vi "Read Static Values.vi"(8 "error in (no error)":errorcluster, 10 "Measurement (0: Current)":u16(ring) items=["Current", "Voltage", "Resistance", "Power", "Temperature", "MPPT Energy"], 11 "VISA resource name":refnum<visa-resource-name>) -> (0 "error out":errorcluster, 2 "Measurement":dbl format="%^#_6g", 3 "VISA resource name out":refnum<visa-resource-name>)   [LabVIEW 2021, in "HH PLI Series.lvlib"]
doc: "Reads static values of current, voltage, resistance, power, instrument temperature and MPPT energy."
uses:
  HH PLI Series.lvlib
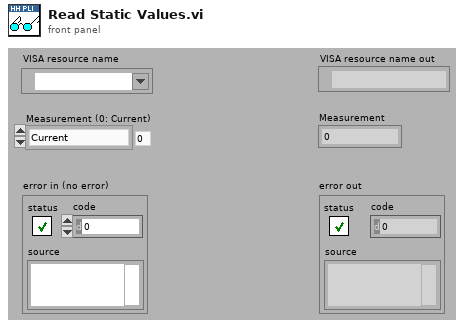
[diagram p1: front panel]
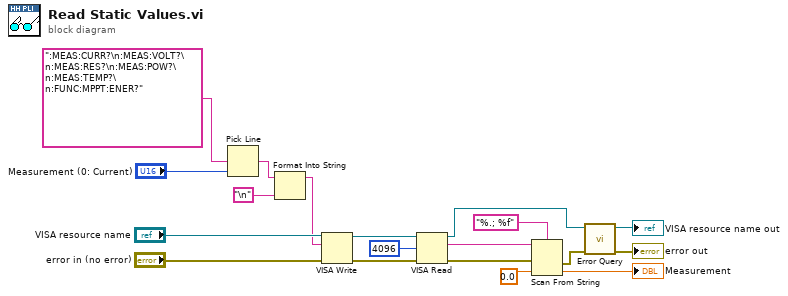
[diagram p0: block diagram]
diagram:
  n1 = Pick Line(multi-line string=":MEAS:CURR?\n:MEAS:VOLT?\n:MEAS:RES?\n:MEAS:POW?\n:MEAS:TEMP?\n:FUNC:MPPT:ENER?", line index="Measurement (0: Current)") -> (output string=w3:string)  [unwired: 1 in]
  n2 = Format Into String(initial string=w3, "\n") -> (resulting string=w1:string)  [unwired: 2 in, 1 out]
  n3 = VISA Write(VISA resource name="VISA resource name", write buffer=w1, error in (no error)="error in (no error)") -> (VISA resource name out=w17:refnum<visa-resource-name>, error out=w16:errorcluster)  [unwired: 1 out]
  n4 = VISA Read(VISA resource name=w17, byte count=u32 4096, error in (no error)=w16) -> (VISA resource name out=w7:refnum<visa-resource-name>, read buffer=w14:string, error out=w12:errorcluster)  [unwired: 1 out]
  n5 = Scan From String(format string="%.; %f", input string=w14, error in=w12, default 1=0.0 ("default value 1")) -> (error out=w6:errorcluster, output 1=→"Measurement":dbl)  [unwired: 1 in, 2 out]
  n6 = call "Error Query.vi"("error in (no error)"=w6, "VISA resource name"=w7) -> ("error out"=→"error out":errorcluster, "VISA resource name out"=→"VISA resource name out":refnum<visa-resource-name>)  [unwired: 6 in, 2 out]
